vi "MicCalibration.vi"(9 "Type":T2(tab)=enum."Voltage", 11 "Settings":T3={"Name of test"="", "Date"=timestamp(3691169924 s since 1904-01-01), "Location"="", "Template"="", "Soundcard"="", "resolution"=32, "Sampling rate"=48000, "Ch1 Gain "=25.0, "Ch2 Gain"=10.0, "Sample time (s)"=0.3, "Pre-trigger (s)"=0.01, "Hammer Threshold"=10.0, "Positions"=12, "Taps/Position"=5, "Set Names"="", "Freq resolution"=10.0, "Hammer cutoff"=0.0, "Mic cutoff"=0.0, "Double bounce "=0.0, "Hammer Cal"=10.0, "dB Offset"=0.0, "Accel Cal"=10.0, "Vibrometer Cal"=0.0, "Mic Cal"=0.0, "Output"=2, "Voltage Cal"=1.0, "Vibrometer Port"="ASRL27::INSTR", "Range"=4, "High Pass"=2, "Bandwidth"=4, "X Range"=[], "Y Range"=[], "dB Spread"=0.0, "Trigger"=0, "Ch_1"=25, "Ch_2"=25, "flip?"=FALSE, "60Hz"=FALSE, "Time offset"=0.0, "Piezo Cal"=1.0, "Default Notes"=""} {"Ch_2" min=1 step=1; "Ch_1" min=1 max=100 step=1; "Trigger" items=["Hammer (force)", "Self-tap", "Spacebar"]; "Bandwidth" items=["1 kHz"=1, "5 kHz"=5, "10 kHz"=10, "25 kHz"=25, "50 kHz"=50, "100 kHz"=100]; "High Pass" items=["Off", "13 Hz", "104 Hz"]; "Range" items=["10 mm/s"=1, "20 mm/s"=2, "50 mm/s"=5, "100 mm/s"=10, "200 mm/s"=20, "500 mm/s"=50, "1 m/s"=100, "2 m/s"=200]; "Output" items=["Accelerometer", "Speed (from acceleration)", "Microphone", "Vibrometer", "Piezo"]; "Voltage Cal" format="%#_13g"; "Ch2 Gain" format="%#_13g"; "Ch1 Gain" format="%#_13g"; "Double bounce" min=0.0; "Mic cutoff" min=0.0 format="%#_4g"; "Hammer cutoff" min=0.0 format="%#_4g"; "Freq resolution" min=0.0; "Pre-trigger (s)" format="%#_13g"; "Date" format="%<%H:%M\n%d/%m/%y>T"; "resolution" items=["16 bit"=16, "24 bit"=24, "32 bit"=32]; "Sampling rate" items=["22050 samp/s"=22050, "44100 samp/s"=44100, "48000 samp/s"=48000]}) -> (3 "Settings Out":T3={"Name of test"="", "Date"=timestamp(0 s since 1904-01-01), "Location"="", "Template"="", "Soundcard"="", "resolution"=32, "Sampling rate"=48000, "Ch1 Gain "=25.0, "Ch2 Gain"=10.0, "Sample time (s)"=0.3, "Pre-trigger (s)"=0.01, "Hammer Threshold"=10.0, "Positions"=12, "Taps/Position"=5, "Set Names"="", "Freq resolution"=10.0, "Hammer cutoff"=0.0, "Mic cutoff"=0.0, "Double bounce "=0.0, "Hammer Cal"=1.0, "dB Offset"=0.0, "Accel Cal"=1.0, "Vibrometer Cal"=1.0, "Mic Cal"=1.0, "Output"=2, "Voltage Cal"=1.0, "Vibrometer Port"="ASRL27::INSTR", "Range"=4, "High Pass"=2, "Bandwidth"=4, "X Range"=[], "Y Range"=[], "dB Spread"=0.0, "Trigger"=0, "Ch_1"=25, "Ch_2"=25, "flip?"=FALSE, "60Hz"=FALSE, "Time offset"=0.0, "Piezo Cal"=1.0, "Default Notes"=""} {"Ch_2" min=1 step=1; "Ch_1" min=1 max=100 step=1; "Trigger" items=["Hammer (force)", "Self-tap", "Spacebar"]; "Bandwidth" items=["1 kHz"=1, "5 kHz"=5, "10 kHz"=10, "25 kHz"=25, "50 kHz"=50, "100 kHz"=100]; "High Pass" items=["Off", "13 Hz", "104 Hz"]; "Range" items=["10 mm/s"=1, "20 mm/s"=2, "50 mm/s"=5, "100 mm/s"=10, "200 mm/s"=20, "500 mm/s"=50, "1 m/s"=100, "2 m/s"=200]; "Output" items=["Accelerometer", "Speed (from acceleration)", "Microphone", "Vibrometer", "Piezo"]; "Voltage Cal" format="%#_13g"; "Ch2 Gain" format="%#_13g"; "Ch1 Gain" format="%#_13g"; "Double bounce" min=0.0; "Mic cutoff" min=0.0 format="%#_4g"; "Hammer cutoff" min=0.0 format="%#_4g"; "Freq resolution" min=0.0; "Pre-trigger (s)" format="%#_13g"; "Date" format="%<%H:%M\n%d/%m/%y>T"; "resolution" items=["16 bit"=16, "24 bit"=24, "32 bit"=32]; "Sampling rate" items=["22050 samp/s"=22050, "44100 samp/s"=44100, "48000 samp/s"=48000]})   [LabVIEW 2022 SP3]
uses:
  PreferencesControl.ctl
  <vilib>/Analysis/baseanly.llb/Mean (DBL).vi
  <vilib>/Analysis/5stat.llb/RMS (DBL).vi
  <extravilib>/ChannelInstances/Lossy Stream-a[.](wfm(dbl))/EndpointRead.vi
  Mic/Mic_Global.vi
  <extravilib>/ChannelInstances/Lossy Stream-a[.](wfm(dbl))/Instantiate.vi
  <extravilib>/ChannelInstances/Tag-a[.](wfm(dbl))/Instantiate.vi
  <extravilib>/ChannelInstances/Lossy Stream-a[.](wfm(dbl))/)Channel.vi
  <resource>/ChannelSupport/_ChannelSupport/WaitIfNeeded.vi
  <extravilib>/ChannelInstances/Tag-a[.](wfm(dbl))/EndpointRead.vi
  <extravilib>/ChannelInstances/Lossy Stream-a[.](wfm(dbl)).lvlib
  <extravilib>/ChannelInstances/Tag-a[.](wfm(dbl)).lvlib
  <vilib>/Analysis/NI_AALPro.lvlib
  <vilib>/Analysis/NI_AALBase.lvlib
panel:
  in  "Import Cal":bool
  in  "Calibrations":T1 {"Microphone (mV/Pa)" format="%0.2f"; "Vibrometer(mV/mm/s)" format="%0.2f"; "Accelerometer (mV/m/s2)" format="%0.2f"; "Voltage (V/au)" format="%0.2f"; "Hammer (N/au)" format="%0.2f"}
  in  "New":bool
  out "p-to-p (units)":dbl format="%0.2f"
  out "p-to-p  (V)":dbl=61.115465517721105 format="%0.4f"
  out "p-to-p  (a.u.)":dbl=61.115465517721105 format="%0.4f"
  in  "Home":bool
  in  "Channel":bool
  in  "OK":bool
  in  "Cancel":bool
  out "RMS (units)":dbl format="%0.2f"
  out "mean a.u.":dbl format="%0.2e"
  out "SPL  (dB)":dbl=61.115465517721105 format="%0.2f"
  out "Peak Freq":dbl=61.115465517721105 format="%0.2f"
  out "RMS  (V)":dbl=61.115465517721105 format="%0.4f"
  out "RMS  (a.u.)":dbl=61.115465517721105 format="%0.4f"
  in  "Sample Time (s)":dbl=1.0
  in  "Ch2 Gain":dbl=25.0 format="%#_13g"
  in  "Ch1 Gain":dbl=25.0 format="%#_13g"
  in  "Units":u16(ring) items=["Raw", "Volts", "Units (Pa, mm/s2)"]
  in  "Calibrator SPL":u16(ring)=94 items=["94 dB"=94, "110 dB"=110, "114 dB"=114, "124 dB"=124]
  in  "Current Cal (mV/Pa)":dbl=48.5
  out "Suggested Cal (mV/Pa)":dbl=90.0 format="%#.2g"
  out "Suggested Slope (V/au)":dbl=3.8 format="%0.2f"
  in  "Current Slope (V/au)":dbl=3.8
  in  "Known RMS Voltage (V)":dbl=0.03536
  in  "Known Acceleration (m/s^2)":dbl=14.14
  out "Calc Peak Accel (mV)":dbl=61.115465517721105 format="%0.4f"
  in  "Current Cal (mV/m/s2)":dbl=1.0
  out "Suggested Cal (mV/m/s2)":dbl=61.115465517721105 format="%0.4f"
  in  "Known RMS velocity (mm/s)":dbl=10.0
  out "RMS Measured (mm/s)":dbl=61.115465517721105 format="%0.4f"
  in  "Current Cal (mV/mm/s)":dbl=1.0
  out "Suggested Cal (mV/mm/s)":dbl=61.115465517721105 format="%0.4f"
  in  "Vibrometer":bool
  in  "Units":bool
  in  "Soundcard":bool
  in  "Microphone":bool
  in  "Accelerometer":bool
  in  "Vibrometer 2":bool
  out "Data":waveform(dbl)(graph)
  out "Spectrum":cluster{dbl, "df":dbl, "FFT {X}":dbl[]}(graph)
  # "Settings"
  # "Channel 1"
  # "Channel 2"
  # "Statistics"
  # "Current Calibration"
  # "Microphone Calibration"
  # "1. Set the calibrator SPL in dB."
  # "2. Turn on the calibrator, which is mounted over the microphone.\n        Make sure you do not have to adjust the gain to keep from clipping"
  # "3. Read and note the \"Suggested Cal\" value."
  # "4. Enter it into the \"Current Cal\" setting."
  # "Soundcard Voltage Calibration"
  # "1. Turn on the voltage source and set the Gain (and channel)."
  # "2. Set the known voltage \n        (I use a sine wave from -50 mV to 50 mV or 35.36mV)."
  # "3. Read and note the \"Suggested Slope\" value."
  # "4. Enter it into the \"Current Slope\" setting."
  # "5. Return to Home to set the sensor calibration."
  # "*Note all measurements are in arbitrary units from the sound card"
  # "Accelerometer Calibration"
  # "1. Turn on the accelerometer calibrator."
  # "2. Set the Known Acceleration in m/s^2"
  # "3. Read and note the \"Suggested Cal\" value."
  # "4. Enter it into the \"Current Cal\" setting."
  # "Vibrometer Calibration"
  # "1. Turn on the vibrometer calibrator and focus the laser on the calibrator."
  # "2. Set the Known RMS velocity in mm/s."
  # "3. Read and note the \"Suggested Cal\" value."
  # "4. Enter it into the \"Current Cal\" setting"
  # "Calibration Wizard"
  # "Instructions at:"
  # "https://sites.google.com/view/oberlinacoustics/software-instructions/calibration-and-units"
  # "You can either calibrate the equipment manually, or test the equipment with the software and calibrate using the recommended values.  Click on what you want to calibrate"
  # "Meaning of the Units"
  # "Calibrating the equiptment and setting these coefficients allow you to process the output in a way that turns raw data, which is in arbitrary units, into more meaningful numbers, in units of Volts, Pascals, Newtons, etc."
  # "On the test screen, you can select the desired units for the Y axis by selecting it from the dropdown menu."
  # "Raw\n\nVolts\n\n\n\nUnits"
  # "Raw data, as it is recorded\n\nChanges the Y axis to show the amplitude in Volts, using the calibration coefficients provided\n\nChanges the Y axis to show amplitude in the most relevant unit (e.g. Pascals for the hammer force), using the calibration coefficients provided"
  # "Hz"
  # "dB"
  # "dB"
  # "sec"
  # "sec"
  # "mV/Pa"
  # "mV/m/s2"
  # "mV/mm/s"
  # "V/N"
  # "sec"
  # "sec"
  # "mV/N"
  # "a.u."
  # "a.u."
  # "sec"
  # "Hz"
  # "dB"
  # "dB"
  # "sec"
  # "sec"
  # "mV/Pa"
  # "mV/m/s2"
  # "mV/mm/s"
  # "V/N"
  # "sec"
  # "sec"
  # "mV/N"
  # "a.u."
  # "a.u."
  # "sec"
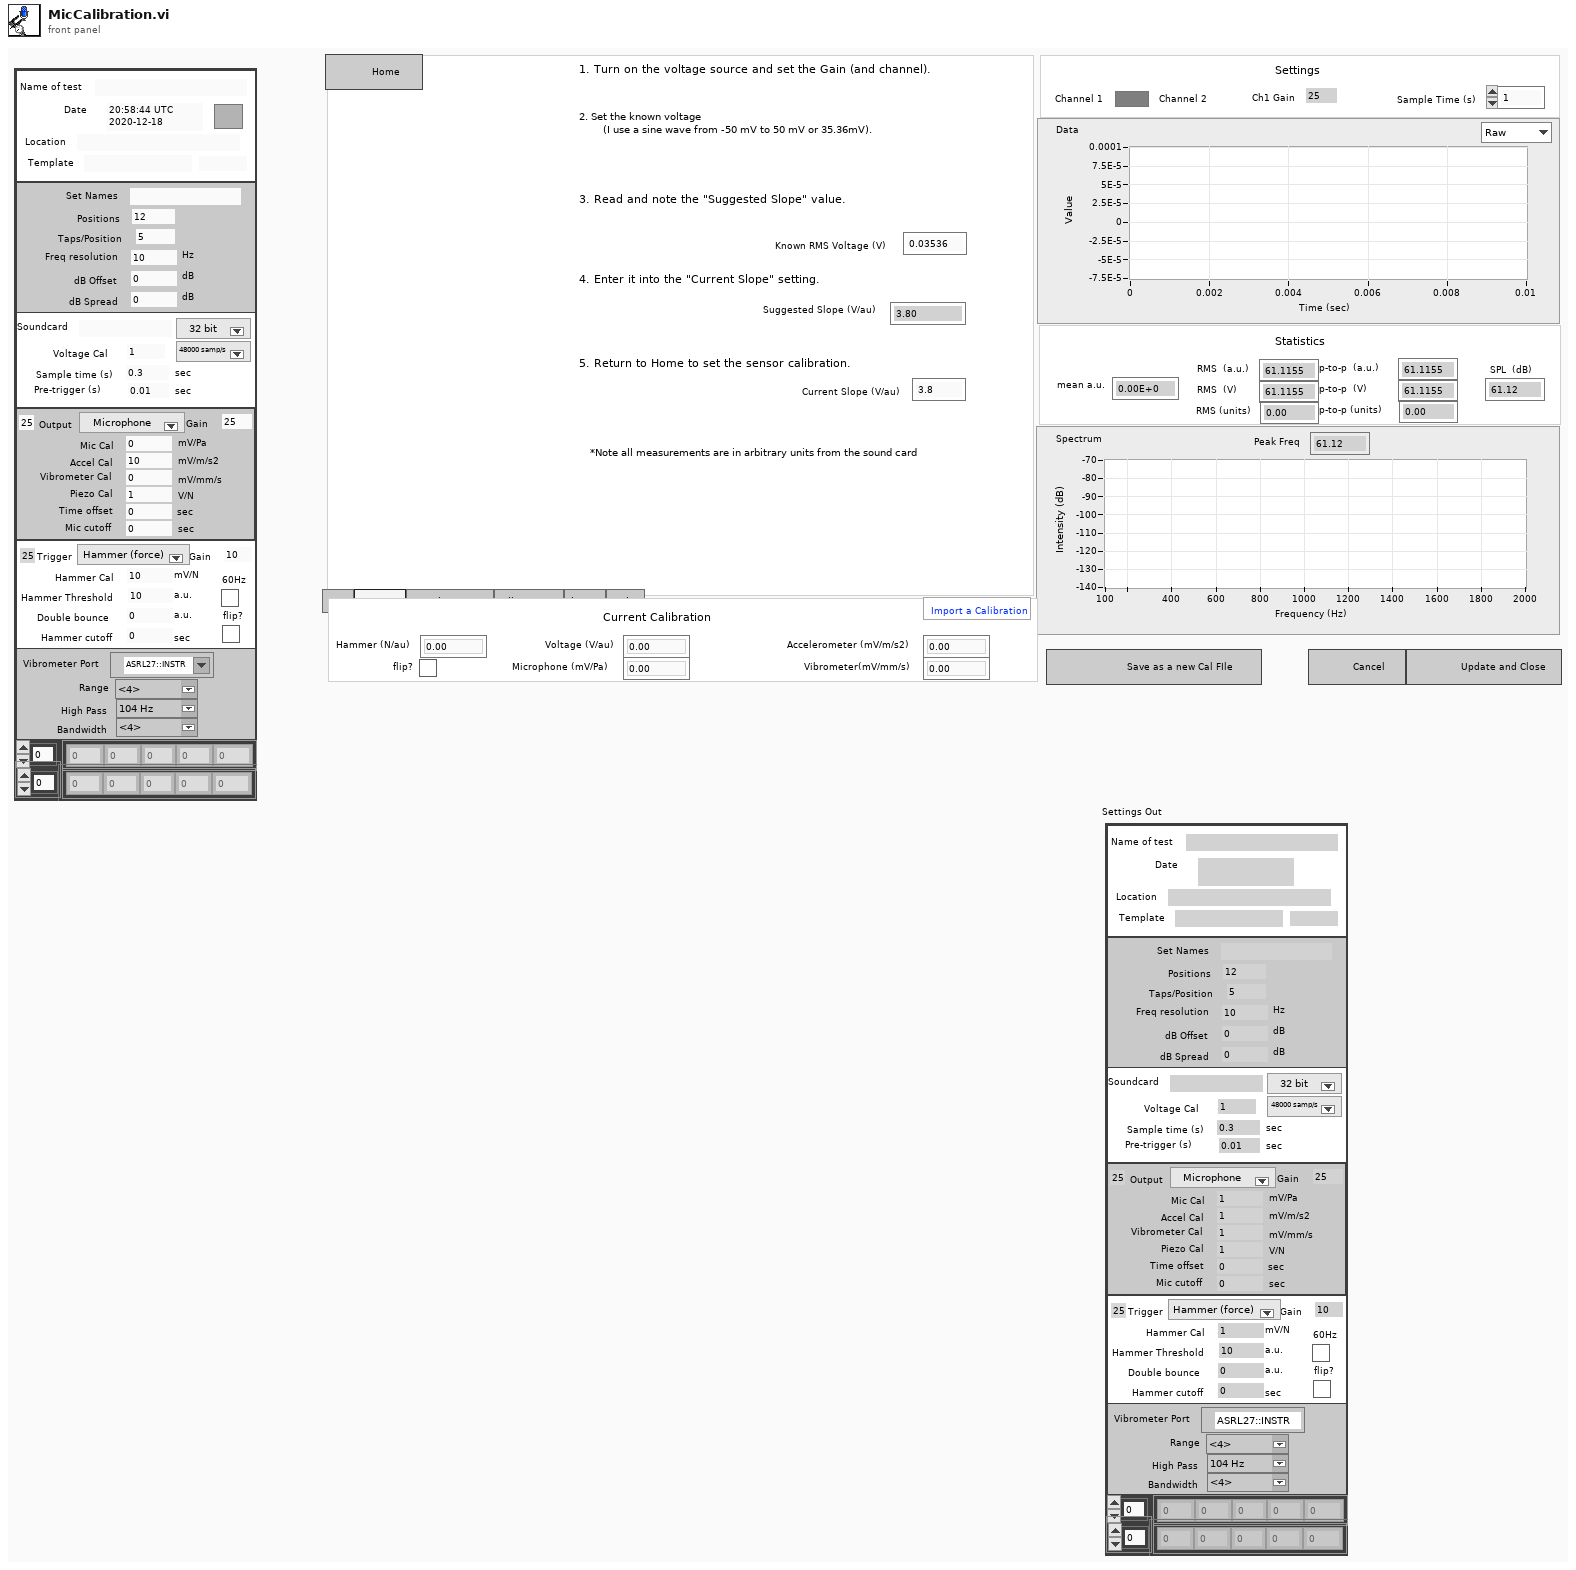
[diagram p1: front panel]
types:
  T1 = cluster{"Hammer (N/au)":dbl, "flip?":bool, "Voltage (V/au)":dbl, "Microphone (mV/Pa)":dbl, "Accelerometer (mV/m/s2)":dbl, "Vibrometer(mV/mm/s)":dbl}
  T2 = enum32{"SPL", "Voltage", "Accelerometer", "Vibrometer", "home", "Units"}
  T3 = typedef "PreferencesControl.ctl" = cluster{"Name of test":string, "Date":timestamp, "Location":string, "Template":string, "Soundcard":string, "resolution":u16, "Sampling rate":u16, "Ch1 Gain ":dbl, "Ch2 Gain":dbl, "Sample time (s)":dbl, "Pre-trigger (s)":dbl, "Hammer Threshold":dbl, "Positions":i16, "Taps/Position":i16, "Set Names":string, "Freq resolution":dbl, "Hammer cutoff":dbl, "Mic cutoff":dbl, "Double bounce ":dbl, "Hammer Cal":dbl, "dB Offset":dbl, "Accel Cal":dbl, "Vibrometer Cal":dbl, "Mic Cal":dbl, "Output":u16, "Voltage Cal":dbl, "Vibrometer Port":refnum<visa-resource-name>, "Range":u16, "High Pass":u16, "Bandwidth":u16, "X Range":cluster{"Minimum":dbl, "Maximum":dbl, "Increment":dbl, "Minor Increment":dbl, "Start":dbl}[], "Y Range":cluster{"Minimum":dbl, "Maximum":dbl, "Increment":dbl, "Minor Increment":dbl, "Start":dbl}[], "dB Spread":dbl, "Trigger":u16, "Ch_1":u8, "Ch_2":u8, "flip?":bool, "60Hz":bool, "Time offset":dbl, "Piezo Cal":dbl, "Default Notes":string}
  T4 = enum16{"Initialize", "Free run", "One Shot - waiting", "One Shot - triggered", "Wait", "Close"}
  T5 = typedef "Tag-a[.](wfm(dbl)).lvlib/))Channel.ctl" = refnum<queue>
  T6 = typedef "Lossy Stream-a[.](wfm(dbl)).lvlib/)Channel.ctl" = refnum<queue>
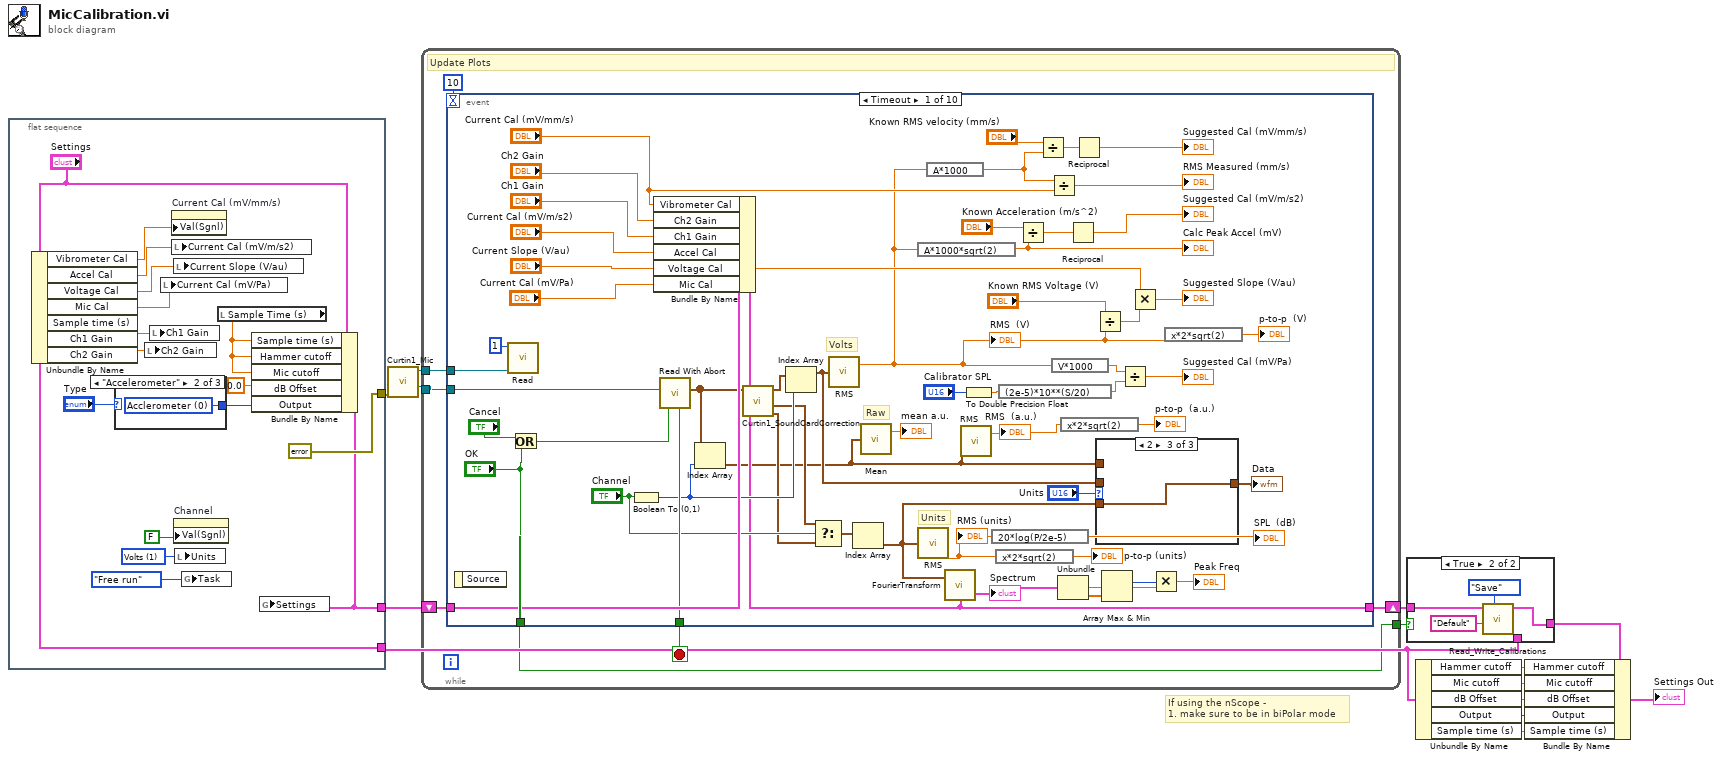
[diagram p0: block diagram]
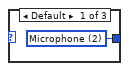
[diagram p3: hidden frame]
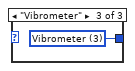
[diagram p4: hidden frame]
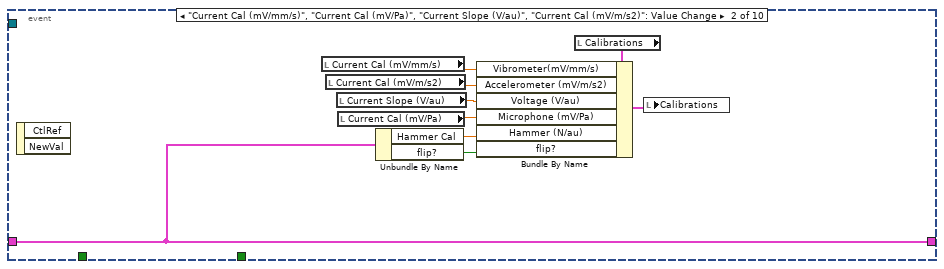
[diagram p7: hidden frame]
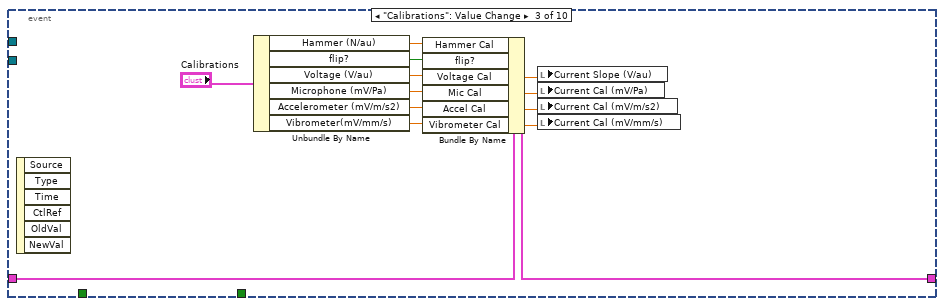
[diagram p8: hidden frame]
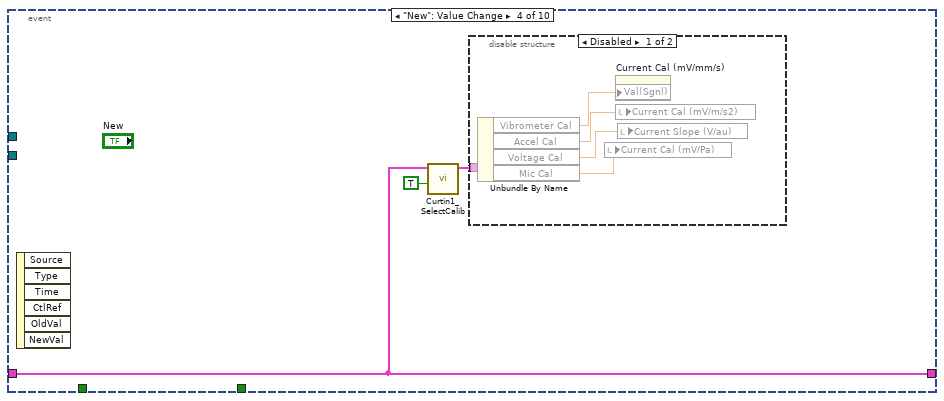
[diagram p9: hidden frame]
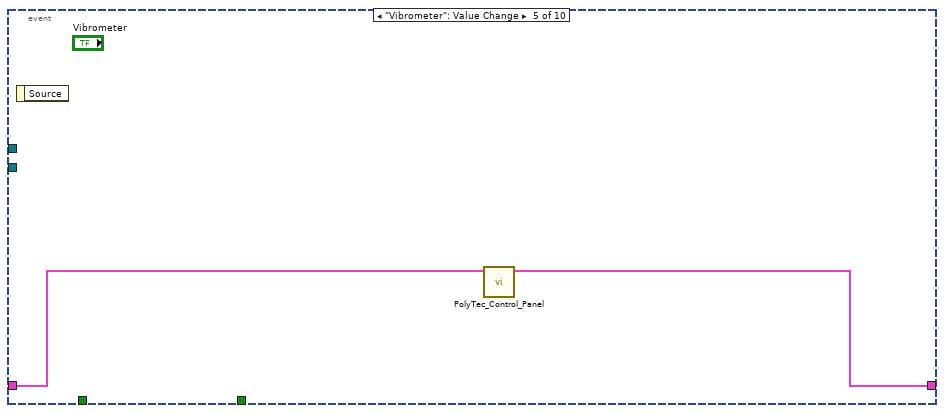
[diagram p11: hidden frame]
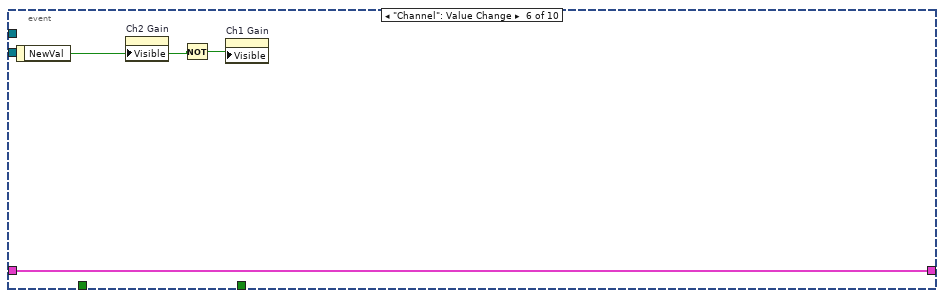
[diagram p12: hidden frame]
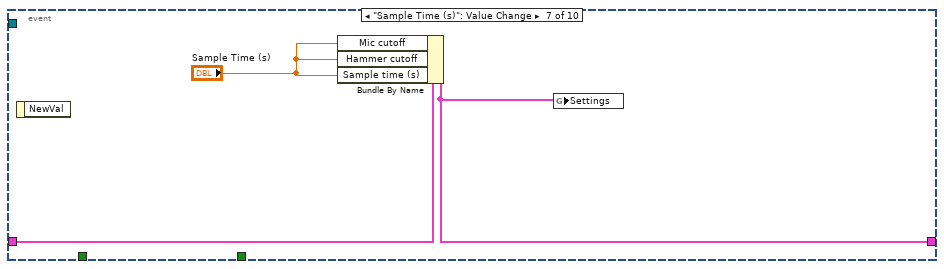
[diagram p13: hidden frame]
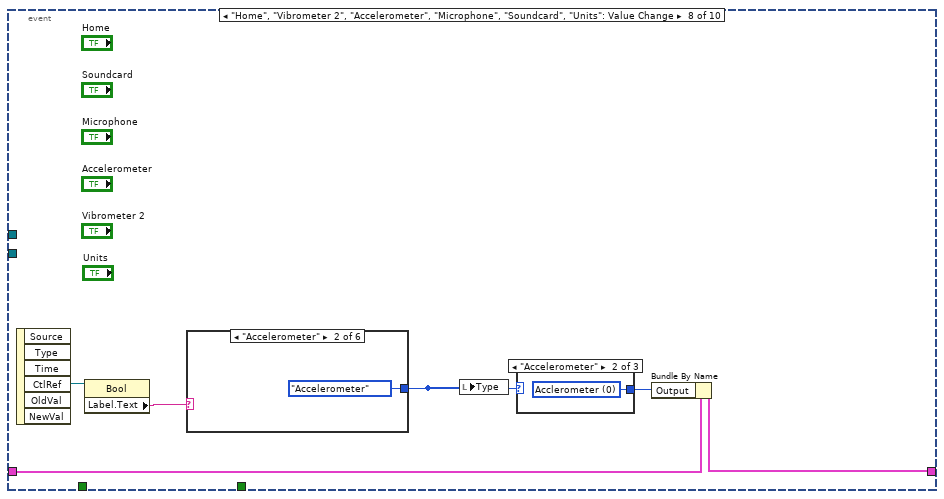
[diagram p14: hidden frame]
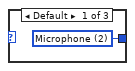
[diagram p15: hidden frame]
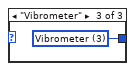
[diagram p16: hidden frame]
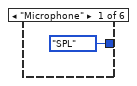
[diagram p17: hidden frame]
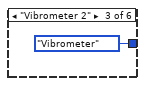
[diagram p18: hidden frame]
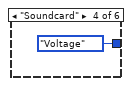
[diagram p19: hidden frame]
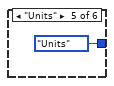
[diagram p20: hidden frame]
diagram:
  # "If using the nScope - \n1. make sure to be in biPolar mode"
  n1 = flat-sequence {
    tunnel: [w18] -> w11
    tunnel: [errorcluster {"status"=FALSE, "code"=0, "source"=""} ("error in (no error)")] -> w14
    tunnel: ["Settings"] -> w10
    frame #0 {
      w27 = u16 1 items=["Raw", "Volts", "Pascal"] ("Units")
      n2 = Unbundle By Name("Settings") -> ("Vibrometer Cal"=w15:dbl, "Accel Cal"=w21:dbl, "Voltage Cal"=w20:dbl, "Mic Cal"=w28:dbl, "Ch1 Gain"=w25:dbl, "Ch2 Gain"=w23:dbl)  [unwired: 1 out]
      n3 = case shown="\"Accelerometer\"" "Type" {
        tunnel: [w31 w32 w33] -> w26
        frame Default {
          w31 = u16 2 items=["Acclerometer", "Displacement", "Microphone", "Vibrometer"] ("Channel 1")
        }
        frame "Accelerometer" {
          w32 = u16 0 items=["Acclerometer", "Displacement", "Microphone", "Vibrometer"] ("Channel 1")
        }
        frame "Vibrometer" {
          w33 = u16 3 items=["Acclerometer", "Displacement", "Microphone", "Vibrometer"] ("Channel 1")
        }
      }
      n4 = local write "Ch2 Gain"(w23) -> ()
      n5 = local write "Ch1 Gain"(w25) -> ()
      n6 = local write "Current Cal (mV/Pa)"(w28) -> ()
      n7 = property on="Current Cal (mV/mm/s)" class="DigNum (strict)"("Val(Sgnl)"=w15) -> ()  [unwired: 2 in, 2 out]
      n8 = local write "Current Cal (mV/m/s2)"(w21) -> ()
      n9 = local write "Current Slope (V/au)"(w20) -> ()
      n10 = property on="Channel" class="Bool (strict)"("Val(Sgnl)"=FALSE ("Channel")) -> ()  [unwired: 2 in, 2 out]
      n11 = local write "Units"(w27) -> ()
      n12 = global write "Mic_Global.vi" "Task"(T4."Free run" ("Task")) -> ()
      n13 = local read "Sample Time (s)"() -> (w17:dbl)
      n14 = Bundle By Name(cluster="Settings", "Sample time (s)"=w17, "Hammer cutoff"=w17, "Mic cutoff"=w17, "dB Offset"=0.0, "Output"=w26) -> (w18:T3)
      n15 = global write "Mic_Global.vi" "Settings"(w18) -> ()
    }
  }
  n16 = call "Curtin1_Mic.vi"("error in (no error)"=w14) -> ("latest data"=w13:T5, "Tap"=w12:T6)  [unwired: 9 in]
  n17 = while {
    tunnel: w13 -> [w40]
    tunnel: w12 -> [w39]
    shift-right: [w35] -> w2
    shift-left: w11 -> [w38]
    tunnel: [w34] -> w1
    stop <- w36 stop-if-true
    # "Update Plots"
    n18 = event shown="[0] Timeout" {
      selector: _ -> [_ _ _ _ _ _ _ _ _ _]
      dyn-events: _ -> [_ _ _ _ _ _ _ _ _ _]
      timeout: 10 -> [_ _ _ _ _ _ _ _ _ _]
      tunnel: w40 -> [w96 _ _ _ _ _ _ _ _ w161]
      tunnel: ["OK" _ _ _ _ _ _ _ _ _] -> w34
      tunnel: w39 -> [w94 _ _ _ _ _ _ _ _ _]
      tunnel: w38 -> [w87 w103 w115 w120 w128 w129 w134 w137 w155 w157]
      tunnel: [w85 _ _ _ _ _ _ _ _ w159] -> w36
      tunnel: [w63 w103 w114 w120 w127 w129 w133 w136 w150 w157] -> w35
      event Timeout {
        # "Units"
        # "Raw"
        # "Volts"
        n19 = event-data() -> ()  [unwired: 1 in, 1 out]
        n20 = call <extravilib>:"Read.vi"("channel"=w94, "timeout in ms (-1)"=1) -> ()  [unwired: 4 in, 6 out]
        n21 = Or(x="Cancel", y="OK") -> (x .or. y?=w95:bool)
        n22 = Boolean To (0,1)(Boolean="Channel") -> (0, 1=w73:i16)
        n23 = Bundle By Name(cluster=w87, "Vibrometer Cal"="Current Cal (mV/mm/s)", "Ch2 Gain"="Ch2 Gain", "Ch1 Gain"="Ch1 Gain", "Accel Cal"="Current Cal (mV/m/s2)", "Voltage Cal"="Current Slope (V/au)", "Mic Cal"="Current Cal (mV/Pa)") -> (w63:T3)
        n24 = call <extravilib>:"Read With Abort.vi"("abort"=w95, "channel"=w96) -> ("element"=w80:waveform(dbl)[], "aborted?"=w85:bool)  [unwired: 7 in, 1 out]
        n25 = Index Array(array=w80, index=w73) -> (element=w55:waveform(dbl))
        n26 = call "Curtin1_SoundCardCorrection.vi"("Settings"=w63, "Buffer in"=w80) -> ("Microphone"=w70:waveform(dbl)[], "Hammer"=w69:waveform(dbl)[], "Volts Out"=w91:waveform(dbl)[])  [unwired: 4 in, 3 out]
        n27 = Index Array(array=w91, index=w73) -> (element=w79:waveform(dbl))
        n28 = Select(t=w69, s="Channel", f=w70) -> (s? t:f=w71:waveform(dbl)[])
        n29 = call-poly <vilib>:"RMS.vi"("X"=w79) -> ("rms value"=w44:dbl)  [unwired: 1 out]
        "RMS  (V)" <- w44
        n30 = Index Array(array=w71) -> (element=w61:waveform(dbl))  [unwired: 1 in]
        n31 = call-poly <vilib>:"Mean.vi"("X"=w55) -> ("mean"=→"mean a.u.":dbl)  [unwired: 1 out]
        n32 = expression code="A*1000*sqrt(2)"(w44) -> (w74:dbl)
        "Calc Peak Accel (mV)" <- w74
        n33 = call-poly <vilib>:"RMS.vi"("X"=w61) -> ("rms value"=w42:dbl)  [unwired: 1 out]
        "RMS (units)" <- w42
        n34 = expression code="A*1000"(w44) -> (w52:dbl)
        n35 = call "FourierTransform.vi"("Settings"=w63, "Data"=w61) -> ("Magnitude of Spectrum"=w60:cluster{"x0":dbl, "df":dbl, dbl[]})  [unwired: 2 in, 1 out]
        "Spectrum" <- w60
        n36 = call-poly <vilib>:"RMS.vi"("X"=w55) -> ("rms value"=w46:dbl)  [unwired: 1 out]
        "RMS  (a.u.)" <- w46
        n37 = To Double Precision Float(number="Calibrator SPL") -> (double precision float=w92:dbl)
        n38 = expression code="20*log(P/2e-5)"(w42) -> (→"SPL  (dB)":dbl)
        n39 = expression code="x*2*sqrt(2)"(w42) -> (→"p-to-p (units)":dbl)
        n40 = expression code="(2e-5)*10**(S/20)"(w92) -> (w89:dbl)
        n41 = Divide(x="Known Acceleration (m/s^2)", y=w74) -> (x/y=w75:dbl)
        n42 = Divide(x="Known RMS velocity (mm/s)", y=w52) -> (x/y=w65:dbl)
        n43 = Divide(x=w52, y="Current Cal (mV/mm/s)") -> (x/y=→"RMS Measured (mm/s)":dbl)
        n44 = expression code="V*1000"(w44) -> (w90:dbl)
        n45 = Unbundle(w60) -> ("df"=w58:dbl, w59:dbl[])  [unwired: 1 out]
        n46 = expression code="x*2*sqrt(2)"(w46) -> (→"p-to-p  (a.u.)":dbl)
        n47 = Reciprocal(x=w75) -> (1/x=→"Suggested Cal (mV/m/s2)":dbl)
        n48 = Reciprocal(x=w65) -> (1/x=→"Suggested Cal (mV/mm/s)":dbl)
        n49 = Divide(x="Known RMS Voltage (V)", y=w44) -> (x/y=w83:dbl)
        n50 = case shown="2" "Units" {
          tunnel: w61 -> [_ _ w100]
          tunnel: [w98 w99 w100] -> w62
          tunnel: w55 -> [w98 _ _]
          tunnel: w79 -> [_ w99 _]
          frame 0, Default {
          }
          frame 1 {
          }
          frame 2 {
          }
        }
        "Data" <- w62
        n51 = Array Max & Min(array=w59) -> (max index (indices)=w57:i32)  [unwired: 3 out]
        n52 = Divide(x=w90, y=w89) -> (x/y=→"Suggested Cal (mV/Pa)":dbl)
        n53 = Multiply(x="Current Slope (V/au)", y=w83) -> (x*y=→"Suggested Slope (V/au)":dbl)
        n54 = Multiply(x=w57, y=w58) -> (x*y=→"Peak Freq":dbl)
        n55 = expression code="x*2*sqrt(2)"(w44) -> (→"p-to-p  (V)":dbl)
      }
      event "Current Cal (mV/mm/s)", "Current Cal (mV/Pa)", "Current Slope (V/au)", "Current Cal (mV/m/s2)": Value Change {
        n56 = event-data() -> ()  [unwired: 1 in, 2 out]
        n57 = local read "Current Cal (mV/mm/s)"() -> (w107:dbl)
        n58 = local read "Current Cal (mV/m/s2)"() -> (w106:dbl)
        n59 = local read "Current Slope (V/au)"() -> (w105:dbl)
        n60 = local read "Current Cal (mV/Pa)"() -> (w104:dbl)
        n61 = Unbundle By Name(w103) -> ("Hammer Cal"=w102:dbl, "flip?"=w101:bool)
        n62 = local read "Calibrations"() -> (w108:T1)
        n63 = Bundle By Name(cluster=w108, "Vibrometer(mV/mm/s)"=w107, "Accelerometer (mV/m/s2)"=w106, "Voltage (V/au)"=w105, "Microphone (mV/Pa)"=w104, "Hammer (N/au)"=w102, "flip?"=w101) -> (w109:T1)
        n64 = local write "Calibrations"(w109) -> ()
      }
      event "Calibrations": Value Change {
        n65 = event-data() -> ()  [unwired: 1 in, 6 out]
        n66 = Unbundle By Name("Calibrations") -> ("Hammer (N/au)"=w118:dbl, "flip?"=w117:bool, "Voltage (V/au)"=w110:dbl, "Microphone (mV/Pa)"=w111:dbl, "Accelerometer (mV/m/s2)"=w112:dbl, "Vibrometer(mV/mm/s)"=w113:dbl)
        n67 = Bundle By Name(cluster=w115, "Hammer Cal"=w118, "flip?"=w117, "Voltage Cal"=w110, "Mic Cal"=w111, "Accel Cal"=w112, "Vibrometer Cal"=w113) -> (w114:T3)
        n68 = local write "Current Slope (V/au)"(w110) -> ()
        n69 = local write "Current Cal (mV/Pa)"(w111) -> ()
        n70 = local write "Current Cal (mV/m/s2)"(w112) -> ()
        n71 = local write "Current Cal (mV/mm/s)"(w113) -> ()
      }
      event "New": Value Change {
        n72 = event-data() -> ()  [unwired: 1 in, 6 out]
        n73 = call "Curtin1_SelectCalib.vi"("Save?"=TRUE ("Update?"), "Settings in"=w120) -> ("Settings out"=w119:T3)  [unwired: 9 in]
        n74 = disable-structure shown="Disabled" {
          disable-tunnel: w119 -> [w122 _]
          frame Disabled {
            n75 = Unbundle By Name(w122) -> ("Vibrometer Cal"=w126:dbl, "Accel Cal"=w124:dbl, "Voltage Cal"=w125:dbl, "Mic Cal"=w123:dbl)
            n76 = local write "Current Cal (mV/Pa)"(w123) -> ()
            n77 = property on="Current Cal (mV/mm/s)" class="DigNum (strict)"("Val(Sgnl)"=w126) -> ()  [unwired: 2 in, 2 out]
            n78 = local write "Current Cal (mV/m/s2)"(w124) -> ()
            n79 = local write "Current Slope (V/au)"(w125) -> ()
          }
          frame Enabled {
          }
        }
      }
      event "Vibrometer": Value Change {
        n80 = event-data() -> ()  [unwired: 1 in, 1 out]
        n81 = call "PolyTec_Control_Panel.vi"("Settings in"=w128) -> ("Settings Out"=w127:T3)  [unwired: 8 in, 2 out]
      }
      event "Channel": Value Change {
        n82 = event-data() -> ("NewVal"=w131:bool)  [unwired: 1 in]
        n83 = property on="Ch2 Gain" class="DigNum (strict)"("Visible"=w131) -> ()  [unwired: 2 in, 2 out]
        n84 = Not(x=w131) -> (.not. x?=w130:bool)
        n85 = property on="Ch1 Gain" class="DigNum (strict)"("Visible"=w130) -> ()  [unwired: 2 in, 2 out]
      }
      event "Sample Time (s)": Value Change {
        n86 = event-data() -> ()  [unwired: 1 in, 1 out]
        n87 = Bundle By Name(cluster=w134, "Mic cutoff"="Sample Time (s)", "Hammer cutoff"="Sample Time (s)", "Sample time (s)"="Sample Time (s)") -> (w133:T3)
        n88 = global write "Mic_Global.vi" "Settings"(w133) -> ()
      }
      event "Home", "Vibrometer 2", "Accelerometer", "Microphone", "Soundcard", "Units": Value Change {
        n89 = event-data() -> ("CtlRef"=w140:refnum<vi>)  [unwired: 1 in, 5 out]
        n90 = property class="Bool"(reference=w140) -> ("Label.Text"=w139:string)  [unwired: 1 in, 2 out]
        n91 = case shown="\"Accelerometer\"" w139 {
          tunnel: [T2."SPL" ("Tyoe") T2."Accelerometer" ("Tyoe") T2."Vibrometer" ("Tyoe") T2."Voltage" ("Tyoe") T2."Units" ("Tyoe") T2."home" ("Tyoe")] -> w135
          frame "Microphone" {
          }
          frame "Accelerometer" {
          }
          frame "Vibrometer 2" {
          }
          frame "Soundcard" {
          }
          frame "Units" {
          }
          frame "Home", Default {
          }
        }
        n92 = local write "Type"(w135) -> ()
        n93 = case shown="\"Accelerometer\"" w135 {
          tunnel: [w141 w142 w143] -> w138
          frame Default {
            w141 = u16 2 items=["Acclerometer", "Displacement", "Microphone", "Vibrometer"] ("Channel 1")
          }
          frame "Accelerometer" {
            w142 = u16 0 items=["Acclerometer", "Displacement", "Microphone", "Vibrometer"] ("Channel 1")
          }
          frame "Vibrometer" {
            w143 = u16 3 items=["Acclerometer", "Displacement", "Microphone", "Vibrometer"] ("Channel 1")
          }
        }
        n94 = Bundle By Name(cluster=w137, "Output"=w138) -> (w136:T3)
      }
      event "Import Cal": Value Change {
        n95 = event-data() -> ()  [unwired: 1 in, 6 out]
        n96 = call "Curtin1_SelectCalib.vi"("Save?"=FALSE ("goal"), "Settings in"=w155) -> ("Settings out"=w150:T3)  [unwired: 9 in]
        n97 = Unbundle By Name(w150) -> ("Vibrometer Cal"=w154:dbl, "Accel Cal"=w152:dbl, "Voltage Cal"=w153:dbl, "Mic Cal"=w151:dbl)
        n98 = local write "Current Cal (mV/Pa)"(w151) -> ()
        n99 = property on="Current Cal (mV/mm/s)" class="DigNum (strict)"("Val(Sgnl)"=w154) -> ()  [unwired: 2 in, 2 out]
        n100 = local write "Current Cal (mV/m/s2)"(w152) -> ()
        n101 = local write "Current Slope (V/au)"(w153) -> ()
      }
      event Panel Close? {
        n102 = event-data() -> ()  [unwired: 1 in, 1 out]
        n103 = call <extravilib>:"Read With Abort.vi"("abort"=TRUE, "channel"=w161) -> ("aborted?"=w159:bool)  [unwired: 7 in, 2 out]
        n104 = event-data("Discard?"=TRUE) -> ()  [unwired: 1 in, 1 out]
      }
    }
  }
  n105 = case shown="True" w1 {
    tunnel: w10 -> [w162 _]
    tunnel: [w162 w165] -> w9
    tunnel: w2 -> [_ w166]
    frame False {
    }
    frame True {
      n106 = call "Read_Write_Calibrations.vi"("Task"=enum16{"Save", "Read", "List"}."Save", "Calibration name"="Default", "Settings in"=w166) -> ("Settings out"=w165:T3)  [unwired: 6 in, 2 out]
    }
  }
  n107 = Unbundle By Name(w10) -> ("Hammer cutoff"=w3:dbl, "Mic cutoff"=w7:dbl, "dB Offset"=w6:dbl, "Output"=w5:u16, "Sample time (s)"=w4:dbl)
  n108 = Bundle By Name(cluster=w9, "Hammer cutoff"=w3, "Mic cutoff"=w7, "dB Offset"=w6, "Output"=w5, "Sample time (s)"=w4) -> (→"Settings Out":T3)
